vi "set_AI_range.vi"(8 "error in (no error)":errorcluster, 9 "Ush.Max":dbl, 10 "U.Max":dbl, 11 "DAQ task (in)":refnum<k21>) -> (0 "error out":errorcluster, 3 "DAQ task (out)":refnum<k21>, 4 "U.Max":dbl, 5 "Ush.Max":dbl, 6 "U.Min":dbl, 7 "Ush.Min":dbl)   [LabVIEW 2017]
uses:
  <resource>/objmgr/daqmx.rc
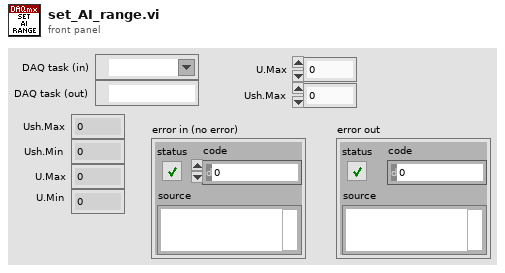
[diagram p1: front panel]
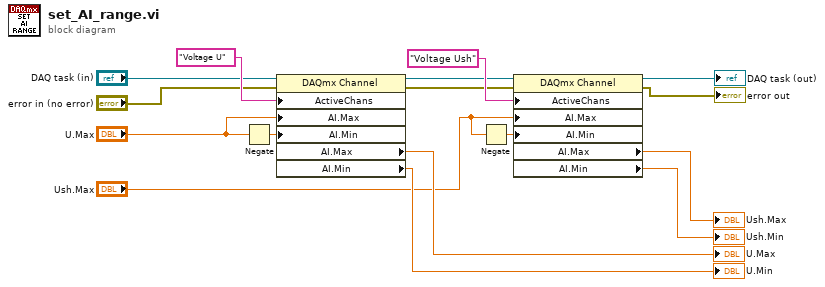
[diagram p0: block diagram]
diagram:
  n1 = Negate(x="U.Max") -> (-x=w4:dbl)
  n2 = property class="DAQmx Channel"(reference="DAQ task (in)", error in="error in (no error)", "ActiveChans"="Voltage U", "AI.Max"="U.Max", "AI.Min"=w4) -> (reference out=w7:refnum<k21>, error out=w8:errorcluster, "AI.Max"=→"U.Max":dbl, "AI.Min"=→"U.Min":dbl)
  n3 = Negate(x="Ush.Max") -> (-x=w2:dbl)
  n4 = property class="DAQmx Channel"(reference=w7, error in=w8, "ActiveChans"="Voltage Ush", "AI.Max"="Ush.Max", "AI.Min"=w2) -> (reference out=→"DAQ task (out)":refnum<k21>, error out=→"error out":errorcluster, "AI.Max"=→"Ush.Max":dbl, "AI.Min"=→"Ush.Min":dbl)
